vi "Record.vi"(8 "error in":errorcluster, 11 "INI file path":path=path "C:/Users/user/Documents/GitHub/AADXB08/AADXB08_LV/data/AADXB08.ini") -> (0 "error out":errorcluster, 1 "Interval":u32, 2 "Trigger_time":string, 3 "Save_day":u32)   [LabVIEW 2019]
uses:
  <vilib>/Utility/config.llb/Read Key (U32).vi
  <vilib>/Utility/config.llb/Read Key (String).vi
  <vilib>/Utility/config.llb/NI_LVConfig.lvlib
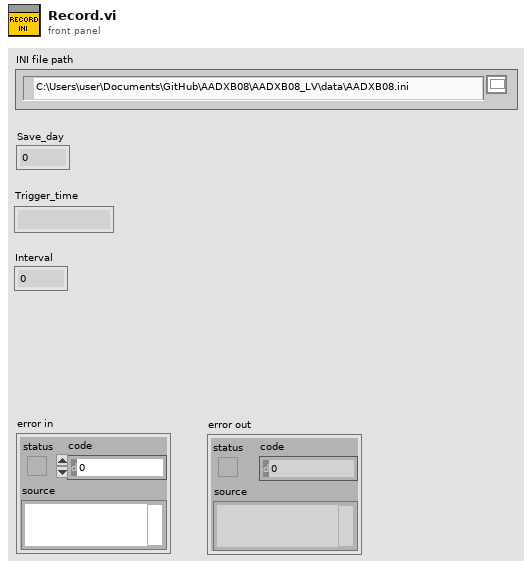
[diagram p1: front panel]
types:
  T1 = typedef "NI_LVConfig.lvlib/Config Data RefNum.ctl" = refnum<k1>
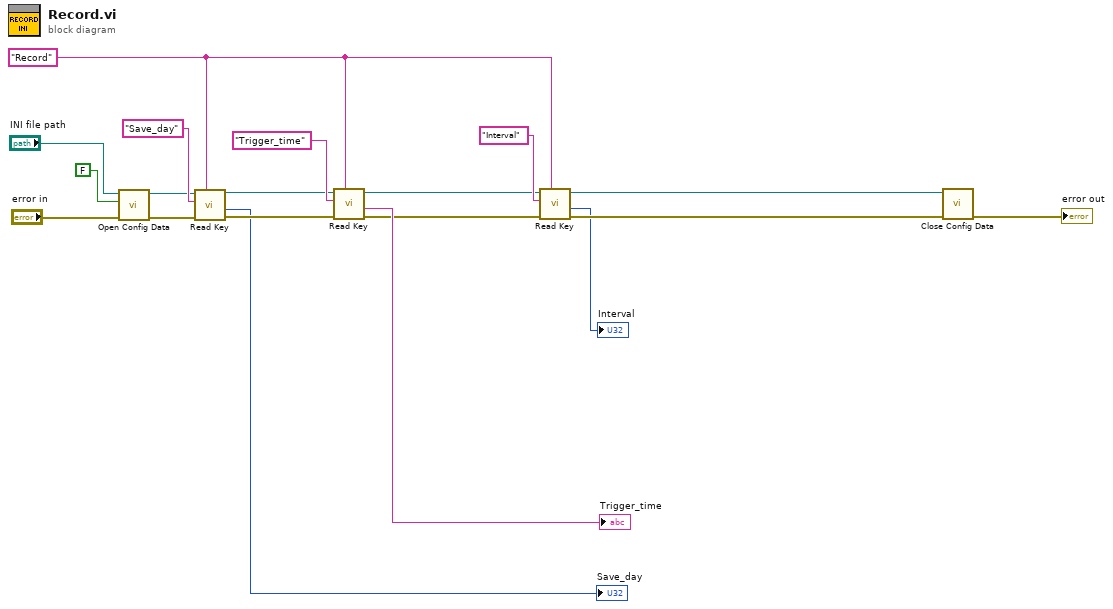
[diagram p0: block diagram]
diagram:
  w4 = "Record" ("Main section")
  n1 = call <vilib>:"Open Config Data.vi"("error in (no error)"="error in", "create file if necessary (T)"=FALSE ("create file if necessary? (T)"), "configuration file path"="INI file path") -> ("error out"=w17:errorcluster, "refnum"=w15:T1)  [unwired: 6 in, 1 out]
  n2 = call-poly <vilib>:"Read Key.vi"("section"=w4, "error in (no error)"=w17, "key"="Save_day", "refnum"=w15) -> ("error out"=w10:errorcluster, "value"=→"Save_day":u32, "refnum out"=w11:T1)  [unwired: 1 in, 4 out]
  n3 = call-poly <vilib>:"Read Key.vi"("section"=w4, "error in (no error)"=w10, "key"="Trigger_time", "refnum"=w11) -> ("error out"=w5:errorcluster, "value"=→"Trigger_time":string, "refnum out"=w6:T1)  [unwired: 2 in, 3 out]
  n4 = call-poly <vilib>:"Read Key.vi"("section"=w4, "error in (no error)"=w5, "key"="Interval", "refnum"=w6) -> ("error out"=w2:errorcluster, "value"=→"Interval":u32, "refnum out"=w3:T1)  [unwired: 1 in, 4 out]
  n5 = call <vilib>:"Close Config Data.vi"("error in (no error)"=w2, "refnum"=w3) -> ("error out"=→"error out":errorcluster)  [unwired: 1 in, 8 out]
